vi "Set function.vi"(6 "Allow reset (false)":bool, 8 "error in":errorcluster, 9 "Initial range (R5)":i32=5 min=0 max=9, 10 "Function (F0 - V DC)":T1(ring), 11 "VISA resource name":refnum<visa-resource-name>) -> (0 "error out":errorcluster, 3 "VISA resource name out":refnum<visa-resource-name>)   [LabVIEW 2020, in "Datron D4xxx.lvlib"]
doc: "This VI sets instrument function (F0 to F5). It also sets initial range before function is cahnged because some functions can't be enabled with autorange.\n\"Allow reset\" means that functiion and its default parameters will be set even if function already selected."
uses:
  Datron D4xxx.lvlib
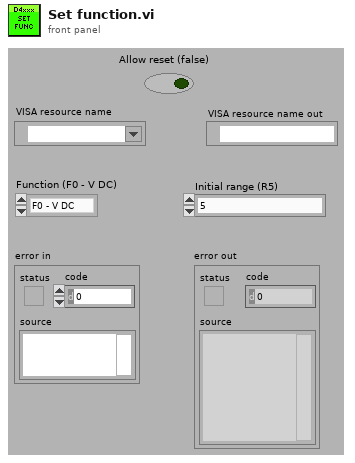
[diagram p1: front panel]
types:
  T1 = enum16{"F0 - V DC", "F1 - V AC", "F2 - A DC", "F3 - A AC", "F4 - R", "F5 - V WB"}
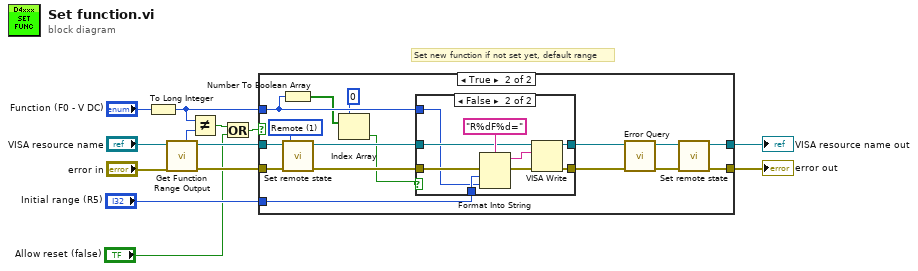
[diagram p0: block diagram]
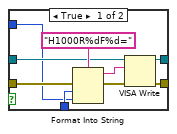
[diagram p3: hidden frame]
diagram:
  # "Set new function if not set yet, default range"
  n1 = To Long Integer(number="Function (F0 - V DC)") -> (32bit integer=w7:i32)
  n2 = call "Get Function Range Output.vi"("error in (no error)"="error in", "VISA resource name"="VISA resource name") -> ("error out"=w11:errorcluster, "VISA resource name out"=w10:refnum<visa-resource-name>, "Function {F0-F5}"=w9:i32)  [unwired: 2 in, 5 out]
  n3 = Not Equal?(x=w7, y=w9) -> (x != y?=w2:bool)
  n4 = Or(x=w2, y="Allow reset (false)") -> (x .or. y?=w3:bool)
  n5 = case shown="True" w3 {
    tunnel: w11 -> [w14 w31]
    tunnel: [w14 w20] -> w4
    tunnel: [w15 w21] -> w5
    tunnel: w10 -> [w15 w30]
    tunnel: w7 -> [_ w19]
    tunnel: "Initial range (R5)" -> [_ w26]
    frame False {
    }
    frame True {
      w27 = u16 1 items=["Local", "Remote", "Default"] ("Remote state")
      n6 = Number To Boolean Array(number=w19) -> (Boolean array=w18:bool[])
      n7 = call "Set remote state.vi"("error in"=w31, "Remote state"=w27, "VISA resource name"=w30) -> ("error out"=w29:errorcluster, "VISA resource name out"=w28:refnum<visa-resource-name>)  [unwired: 7 in]
      n8 = Index Array(array=w18, index=0) -> (element=w16:bool)
      n9 = case shown="False" w16 {
        tunnel: w29 -> [w37 w46]
        tunnel: w28 -> [w36 w45]
        tunnel: w19 -> [w32 w41]
        tunnel: w26 -> [w35 w44]
        tunnel: [w34 w43] -> w23
        tunnel: [w33 w42] -> w22
        frame True {
          n10 = Format Into String(format string="H1000R%dF%d=", error in=w37, w35, w32) -> (resulting string=w40:string, error out=w39:errorcluster)  [unwired: 1 in]
          n11 = VISA Write(VISA resource name=w36, write buffer=w40, error in (no error)=w39) -> (VISA resource name out=w33:refnum<visa-resource-name>, error out=w34:errorcluster)  [unwired: 1 out]
        }
        frame False {
          n12 = Format Into String(format string="R%dF%d=", error in=w46, w44, w41) -> (resulting string=w49:string, error out=w48:errorcluster)  [unwired: 1 in]
          n13 = VISA Write(VISA resource name=w45, write buffer=w49, error in (no error)=w48) -> (VISA resource name out=w42:refnum<visa-resource-name>, error out=w43:errorcluster)  [unwired: 1 out]
        }
      }
      n14 = call "Error Query.vi"("error in (no error)"=w23, "VISA resource name"=w22) -> ("error out"=w25:errorcluster, "VISA resource name out"=w24:refnum<visa-resource-name>)  [unwired: 6 in, 2 out]
      n15 = call "Set remote state.vi"("error in"=w25, "VISA resource name"=w24) -> ("error out"=w20:errorcluster, "VISA resource name out"=w21:refnum<visa-resource-name>)  [unwired: 8 in]
    }
  }
  "VISA resource name out" <- w5
  "error out" <- w4
